vi "Convert Variant To Property.vi"(8 "error in":errorcluster, 11 "Property Variant":variant) -> (0 "error out":errorcluster, 3 "Property Ref out":refnum<data-value>)   [LabVIEW 2024, in "Config File Parser.lvlib" / "Property.lvclass"]
uses:
  Property.lvclass
  Property.lvclass/Property.ctl
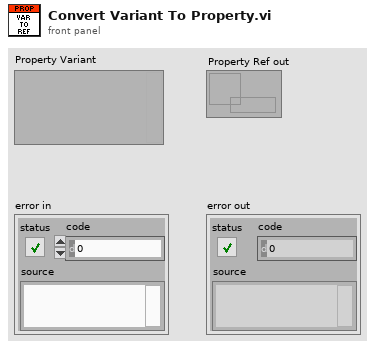
[diagram p1: front panel]
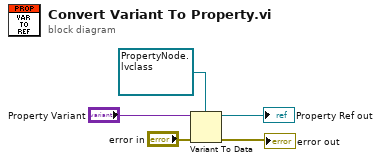
[diagram p0: block diagram]
diagram:
  n1 = Variant To Data(error in="error in", type=refnum<data-value> refnum ("data value reference"), Variant="Property Variant") -> (data=→"Property Ref out":refnum<data-value>, error out=→"error out":errorcluster)
